vi "_U64ToU8Array.vi"(11 "U64In":u64) -> (3 "ArrayOut":u8[](array[numeric]))   [LabVIEW 2018, in "Modbus_Processing_Unit.lvlib" / "MPU.lvclass"]
uses:
  MPU.lvclass
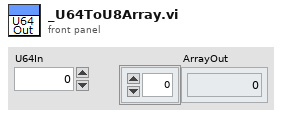
[diagram p1: front panel]
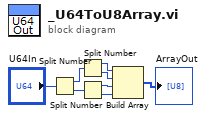
[diagram p0: block diagram]
diagram:
  n1 = Split Number(x="U64In") -> (hi(x)=w1:u32, lo(x)=w2:u32)
  n2 = Split Number(x=w1) -> (hi(x)=w4:u16, lo(x)=w5:u16)
  n3 = Split Number(x=w2) -> (hi(x)=w6:u16, lo(x)=w7:u16)
  n4 = Build Array(w4, w5, w6, w7) -> (→"ArrayOut":u16[])
